vi "Resistance_Single.vi"() -> ()   [LabVIEW 2016]
uses:
  <instrlib>/Keithley 24XX/Public/Data/Read (Single Point).vi
  <instrlib>/Keithley 24XX/Keithley 24XX.lvlib
panel:
  in  "Delay Time (s)":dbl=1.0
  in  "Range(ohm)":u16(ring) items=["AUTO", "2", "2O", "200", "2k", "20k", "200k", "2M", "20M", "200M"]
  in  "2 Wire(F) / 4 Wire(T)":bool
  out "Resistance":sgl=20681.49
  out "Current":sgl=1.000047e-05
  out "Voltage":sgl=0.2068247
  in  "VISA resource name":refnum<visa-resource-name>="COM5"
  # "keithley 24XX source meter series\nHardware settings with RS-232\nMENU->COMMUNICATION->RS-232->Terminator-><LF>\n\n4-wire resistance sensing mode:\nV Source: 4-wire Sense\nI Source: Input/Output"
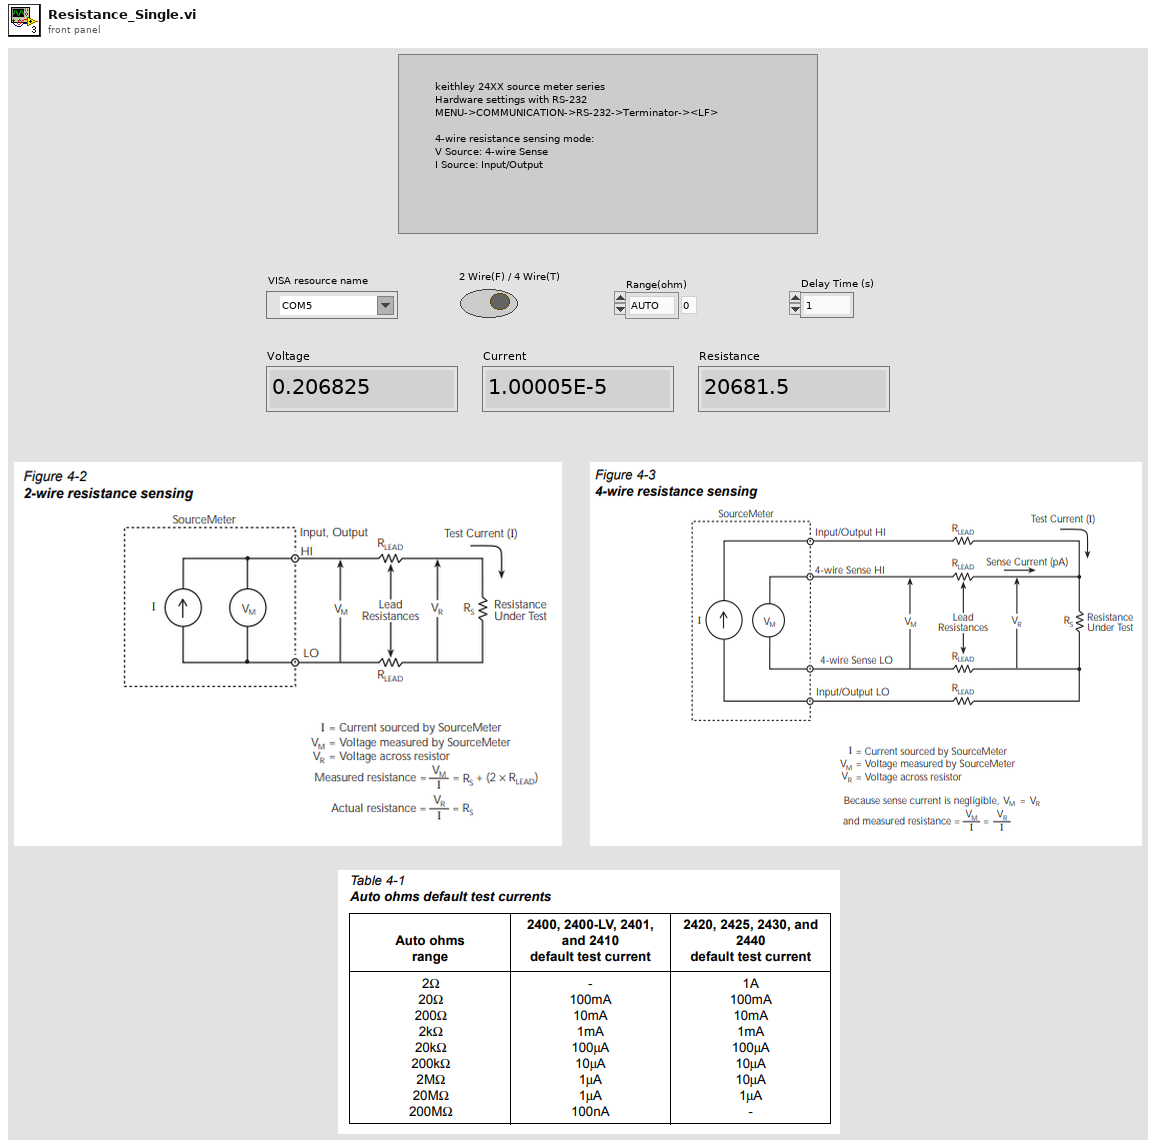
[diagram p1: front panel]
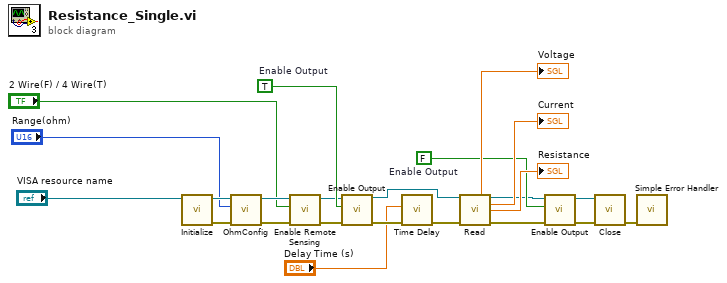
[diagram p0: block diagram]
diagram:
  w13 = TRUE  # Enable Output
  w18 = FALSE  # Enable Output
  n1 = call <instrlib>:"Initialize.vi"("VISA resource name"="VISA resource name") -> ("error out"=w8:errorcluster, "VISA resource name out"=w10:refnum<visa-resource-name>)  [unwired: 9 in]
  n2 = call "OhmConfig.vi"("error in (no error)"=w8, "Function (0: Volts)"="Range(ohm)", "VISA resource name"=w10) -> ("error out"=w7:errorcluster, "VISA resource name out"=w9:refnum<visa-resource-name>)  [unwired: 7 in]
  n3 = call <instrlib>:"Enable Remote Sensing.vi"("error in (no error)"=w7, "Enable Remote Sensing (T: Enable)"="2 Wire(F) / 4 Wire(T)", "VISA resource name"=w9) -> ("error out"=w11:errorcluster, "VISA resource name out"=w12:refnum<visa-resource-name>)  [unwired: 7 in]
  n4 = call <instrlib>:"Enable Output.vi"("error in (no error)"=w11, "Enable Output (T: Enable)"=w13, "VISA resource name"=w12) -> ("error out"=w4:errorcluster, "VISA resource name out"=w2:refnum<visa-resource-name>)  [unwired: 7 in]
  n5 = call "Time Delay"("error in (no error)"=w4, "Delay Time (s)"="Delay Time (s)") -> ("error out"=w3:errorcluster)  [unwired: 9 in]
  n6 = call-poly <instrlib>:"Read.vi"("VISA resource name"=w2, "error in (no error)"=w3) -> ("Voltage"=→"Voltage":sgl, "VISA resource name out"=w14:refnum<visa-resource-name>, "Current"=→"Current":sgl, "Resistance"=→"Resistance":sgl, "error out"=w15:errorcluster)  [unwired: 7 in, 2 out]
  n7 = call <instrlib>:"Enable Output.vi"("error in (no error)"=w15, "Enable Output (T: Enable)"=w18, "VISA resource name"=w14) -> ("error out"=w16:errorcluster, "VISA resource name out"=w17:refnum<visa-resource-name>)  [unwired: 7 in]
  n8 = call <instrlib>:"Close.vi"("error in (no error)"=w16, "VISA resource name"=w17) -> ("error out"=w23:errorcluster)  [unwired: 9 in]
  n9 = call <vilib>:"Simple Error Handler.vi"("error in (no error)"=w23) -> ()  [unwired: 4 in, 5 out]
